vi "RandomNumberSequence.vi"() -> ()   [LabVIEW 2011]
panel:
  out "Waveform Chart 2":dbl[](graph)
  in  "Boolean 2":bool
  # "Generarea De Siruri De Numere Aleatoare"
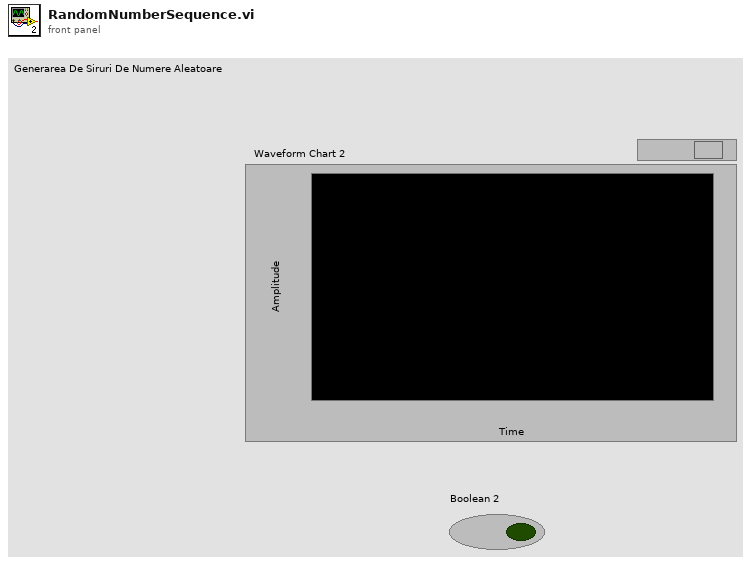
[diagram p1: front panel]
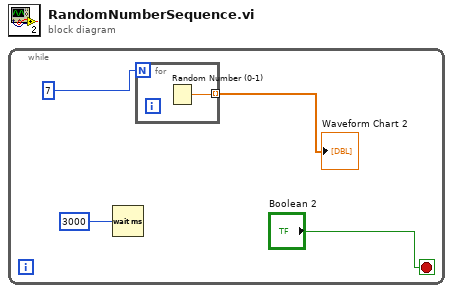
[diagram p0: block diagram]
diagram:
  n1 = while {
    stop <- "Boolean 2" stop-if-true
    n2 = Wait (ms)(milliseconds to wait=3000) -> ()  [unwired: 1 out]
    n3 = for {
      N: 7 -> [_]
      tunnel: [w5] -> w2 mode=indexing
      n4 = Random Number (0-1)() -> (number: 0 to 1=w5:dbl)
    }
    "Waveform Chart 2" <- w2
  }
